vi "lightsource-write.vi"(0 "VISA in":refnum<visa-resource-name>, 2 "set parameters":bool, 3 "NKT Input":T2={"Emission"=FALSE, "Operation Mode"=FALSE, "Power Level"=5.0, "Feedback Level"=0.0, "Short Wavelength (nm)"=560.0, "Long Wavelength (nm)"=580.0, "UV Wavelength (nm)"=400.0} {"UV Wavelength (nm)" min=350.0 max=480.0 step=1.0 format="%.1f"; "Long Wavelength (nm)" min=400.0 max=850.0 step=0.5 format="%.1f"; "Short Wavelength (nm)" min=400.0 max=850.0 step=0.5 format="%.1f"; "Feedback Level" min=0.0 max=90.0 step=0.1 format="%.1f%%"; "Power Level" min=5.0 max=100.0 step=0.1 format="%.1f%%"}) -> (1 "VISA out":refnum<visa-resource-name>, 4 "NKT Output":T1 {"UV Wavelength (nm)" format="%.1f"; "Long Wavelength (nm)" format="%.1f"; "Short Wavelength (nm)" format="%.1f"; "Feedback Level" format="%.1f%%"; "Power Level" format="%.1f%%"; "Temp (°C)" format="%.1f"}, 8 "External Control Cluster":T3)   [LabVIEW 2015]
panel:
  out "Emission on?":bool
  out "Long Wavelength":i32
  out "Short Wavelength":i32
  out "Power Level":i32
  out "Operation Mode":i32
  out "Feedback Level":i32
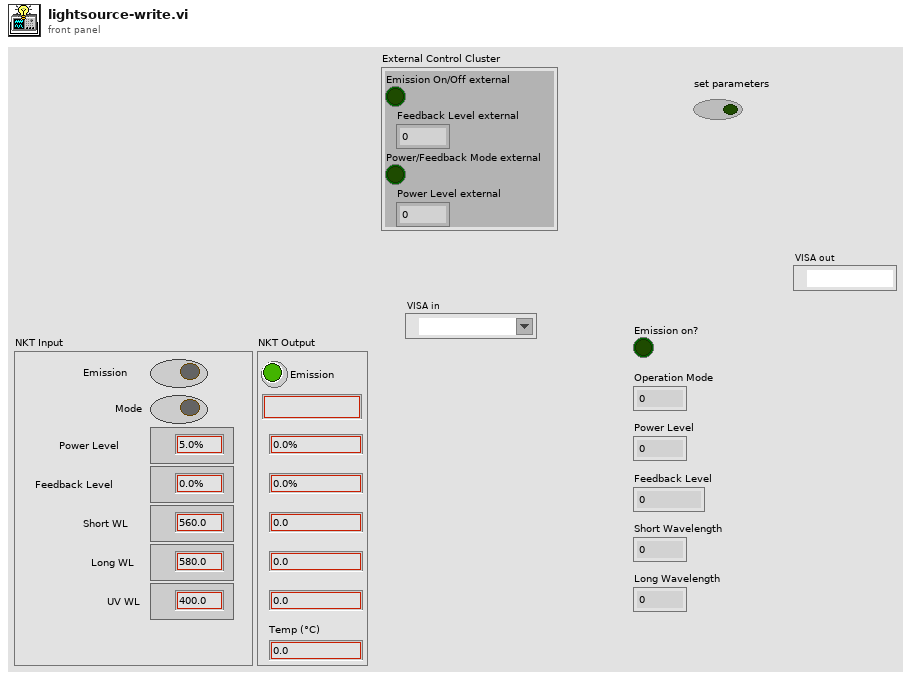
[diagram p1: front panel]
types:
  T1 = cluster{"Emission":bool, "Operation Mode":string, "Power Level":dbl, "Feedback Level":dbl, "Short Wavelength (nm)":dbl, "Long Wavelength (nm)":dbl, "UV Wavelength (nm)":dbl, "Temp (°C)":dbl}
  T2 = cluster{"Emission":bool, "Operation Mode":bool, "Power Level":dbl, "Feedback Level":dbl, "Short Wavelength (nm)":dbl, "Long Wavelength (nm)":dbl, "UV Wavelength (nm)":dbl}
  T3 = cluster{"Emission On/Off external":bool, "Feedback Level external":dbl, "Power/Feedback Mode external":bool, "Power Level external":dbl}
  T4 = cluster{"OpenPort":bool, "ClosePort":bool, "Baudrate":i32, "Wait":u16, "ReadWrite":bool}
  T5 = cluster{"Destination":u8, "Source":u8, "Register":u8, "Array":i16[], "WriteNotRead":bool, "ReadWithPreample":bool, "Ring":u16, "String":string, "Long":i32}
  T6 = cluster{"Source":u8, "TelegramType":u8, "Register":u8, "Destination":u8, "TelegramReceived":bool, "CRC error":bool, "PayloadByteArray":u8[], "(hi.lo)":u16, "Crc16":u16, "Long":i32, "PayloadIntArray":u16[], "String":string}
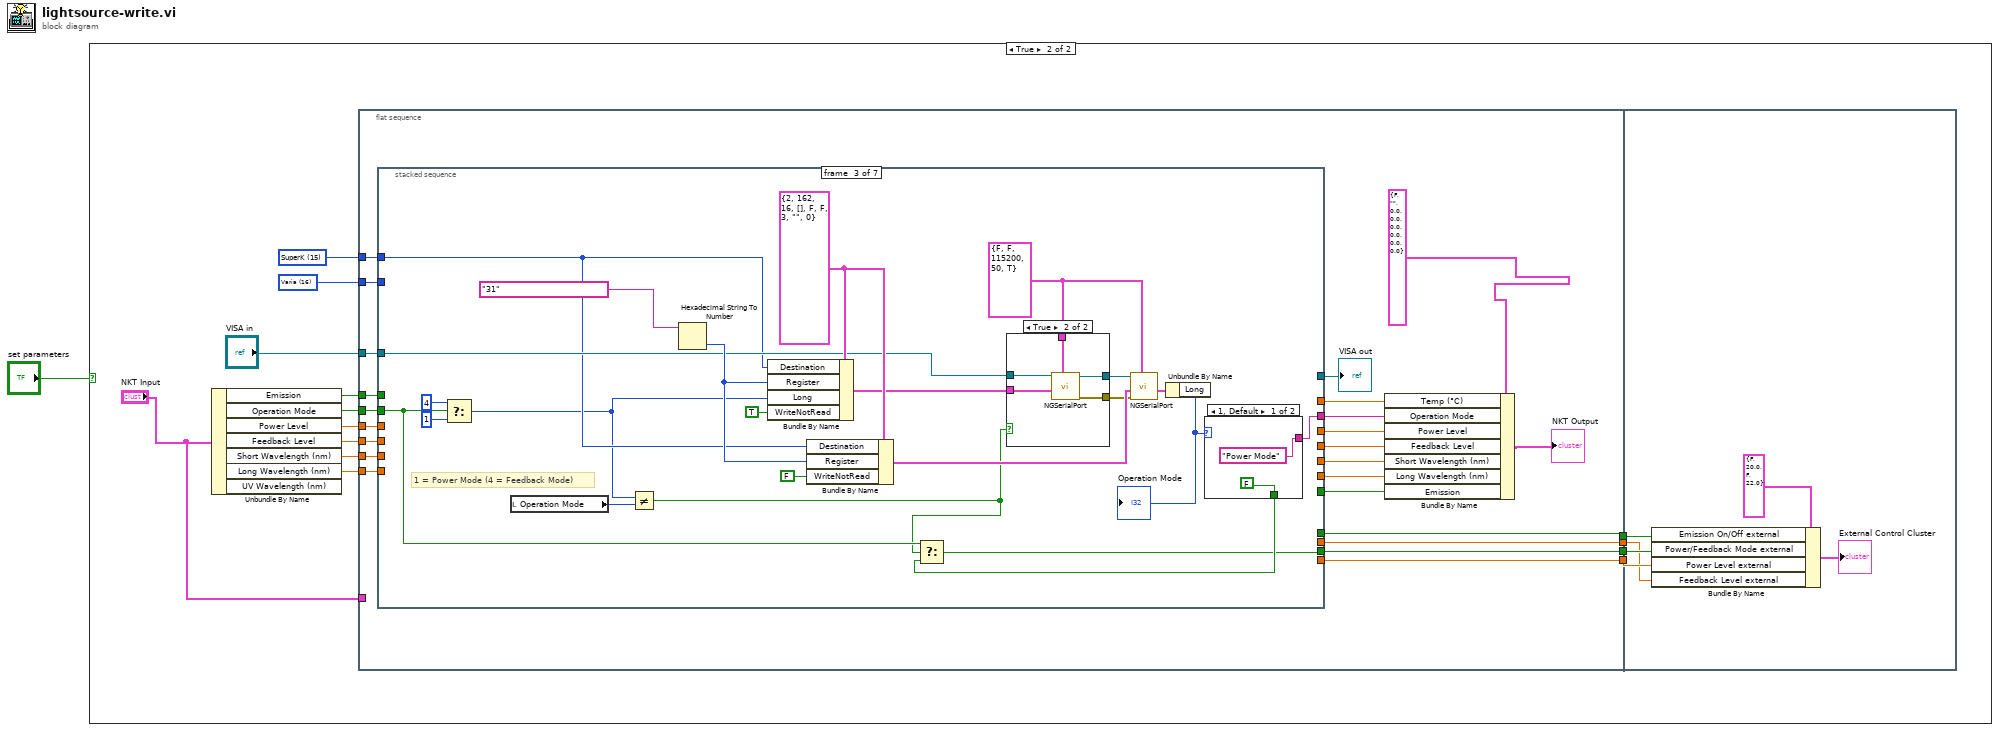
[diagram p0: block diagram]
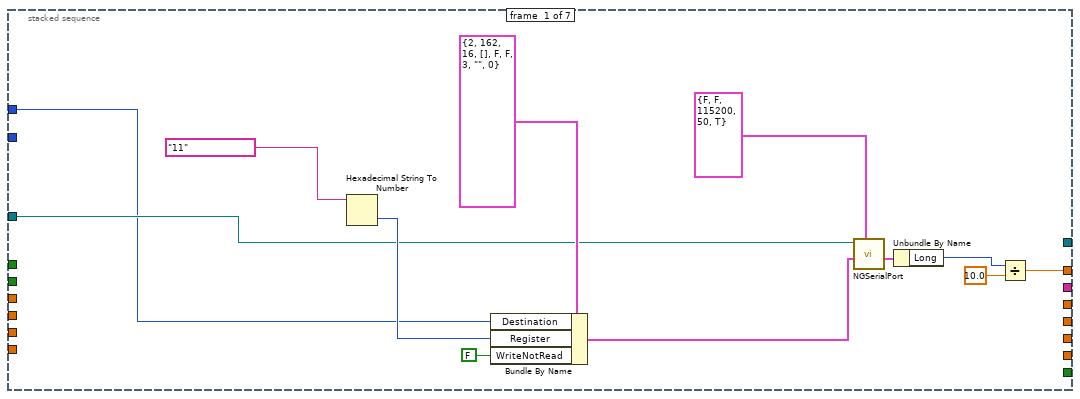
[diagram p3: hidden frame]
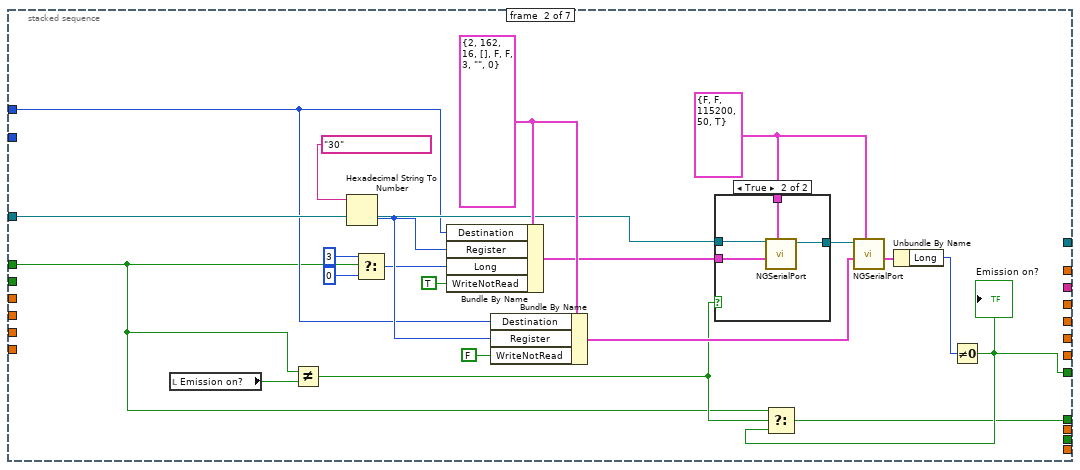
[diagram p4: hidden frame]
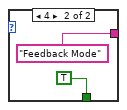
[diagram p6: hidden frame]
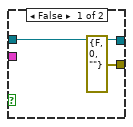
[diagram p7: hidden frame]
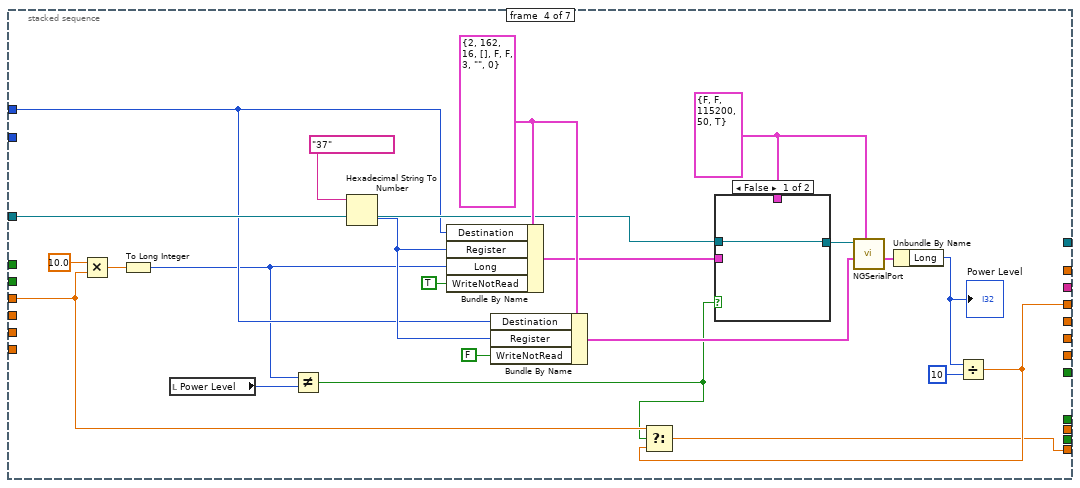
[diagram p8: hidden frame]
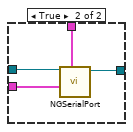
[diagram p9: hidden frame]
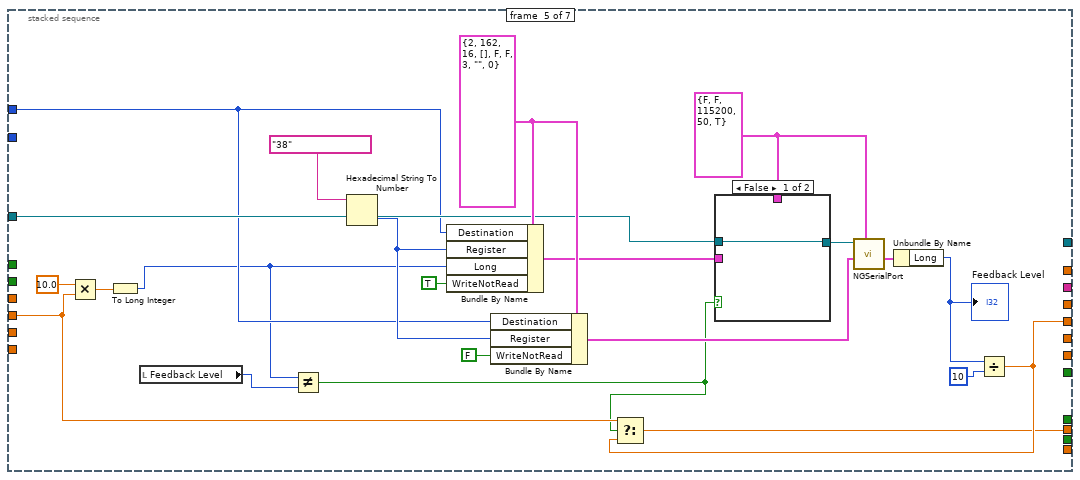
[diagram p10: hidden frame]
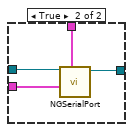
[diagram p11: hidden frame]
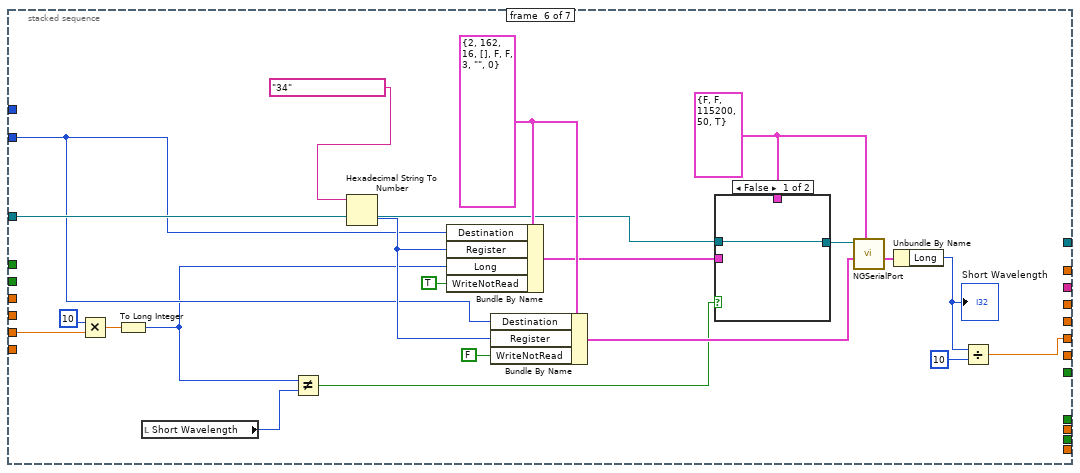
[diagram p12: hidden frame]
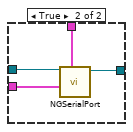
[diagram p13: hidden frame]
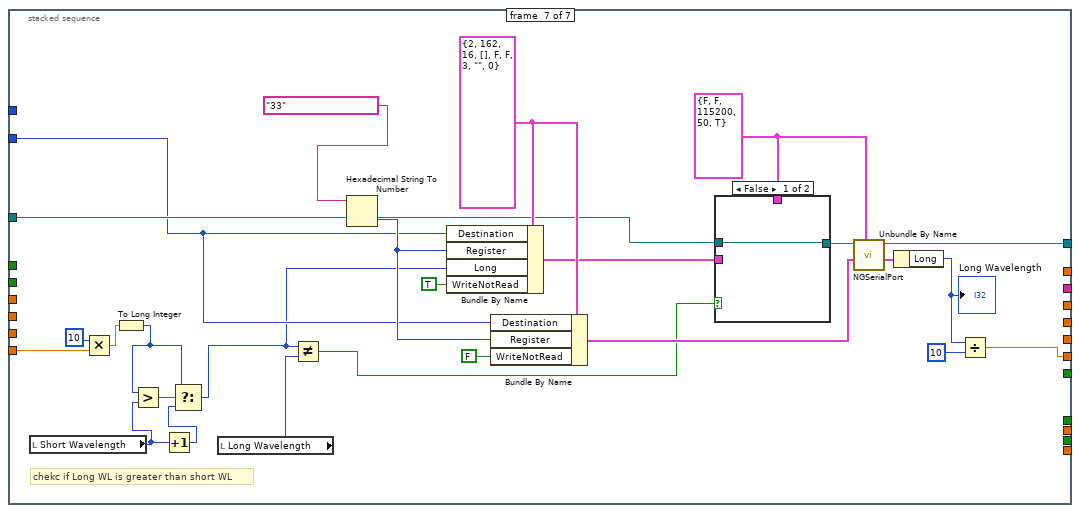
[diagram p14: hidden frame]
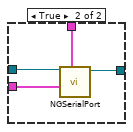
[diagram p15: hidden frame]
diagram:
  n1 = case shown="True" "set parameters" {
    frame False {
    }
    frame True {
      w3 = u16 15 items=["SuperK"=15, "Varia"=16, "UV"=30] ("Module 9")
      w4 = u16 16 items=["SuperK"=15, "Varia"=16, "UV"=30] ("Module 9")
      n2 = Unbundle By Name("NKT Input") -> ("Emission"=w10:bool, "Operation Mode"=w9:bool, "Power Level"=w8:dbl, "Feedback Level"=w7:dbl, "Short Wavelength (nm)"=w6:dbl, "Long Wavelength (nm)"=w5:dbl)  [unwired: 1 out]
      n3 = flat-sequence {
        tunnel: "VISA in" -> [w38]
        tunnel: w3 -> [w36]
        tunnel: w4 -> [w35]
        tunnel: w10 -> [w34]
        tunnel: w9 -> [w33]
        tunnel: w8 -> [w32]
        tunnel: w7 -> [w31]
        tunnel: w6 -> [w30]
        tunnel: w5 -> [w29]
        tunnel: "NKT Input" -> [_]
        tunnel: [w22] -> w15
        tunnel: [w21] -> w14
        tunnel: [w20] -> w13
        tunnel: [w19] -> w12
        tunnel: w15 -> [w226]
        tunnel: w14 -> [w225]
        tunnel: w13 -> [w224]
        tunnel: w12 -> [w227]
        frame #0 {
          n4 = stacked-sequence {
            tunnel: w38 -> [w43 w61 w89 w122 w148 w176 w207]
            tunnel: [_ _ _ _ _ _ w198] -> w37
            tunnel: w36 -> [w42 w60 w88 w121 w147 _ _]
            tunnel: w35 -> [_ _ _ _ _ w175 w206]
            tunnel: [w39 _ _ _ _ _ _] -> w28
            tunnel: w34 -> [_ w54 _ _ _ _ _]
            tunnel: [_ w57 _ _ _ _ _] -> w18
            tunnel: w33 -> [_ _ w81 _ _ _ _]
            tunnel: [_ _ w83 _ _ _ _] -> w27
            tunnel: w32 -> [_ _ _ w114 _ _ _]
            tunnel: [_ _ _ w113 _ _ _] -> w26
            tunnel: w31 -> [_ _ _ _ w141 _ _]
            tunnel: w30 -> [_ _ _ _ _ w169 _]
            tunnel: w29 -> [_ _ _ _ _ _ w200]
            tunnel: [_ _ _ _ w140 _ _] -> w25
            tunnel: [_ _ _ _ _ w165 _] -> w24
            tunnel: [_ _ _ _ _ _ w191] -> w23
            tunnel: [_ _ w79 _ _ _ _] -> w22
            tunnel: [_ _ _ w112 _ _ _] -> w21
            tunnel: [_ _ _ _ w139 _ _] -> w20
            tunnel: [_ w56 _ _ _ _ _] -> w19
            frame #0 {
              n5 = Hexadecimal String To Number(string="11" ("Super K Register 4")) -> (number=w48:u32)  [unwired: 2 in, 1 out]
              n6 = Bundle By Name(cluster=T5 {"Destination"=2, "Source"=162, "Register"=16, "Array"=[], "WriteNotRead"=FALSE, "ReadWithPreample"=FALSE, "Ring"=3, "String"="", "Long"=0} ("InParameters"), "Destination"=w42, "Register"=w48, "WriteNotRead"=FALSE) -> (w47:T5)
              n7 = call "NGSerialPort.vi"("PortParameters"=T4 {"OpenPort"=FALSE, "ClosePort"=FALSE, "Baudrate"=115200, "Wait"=50, "ReadWrite"=TRUE}, "InParameters"=w47, "VISA in"=w43) -> ("OutParameters"=w49:T6)  [unwired: 6 in, 2 out]
              n8 = Unbundle By Name(w49) -> ("Long"=w40:i32)
              n9 = Divide(x=w40, y=10.0) -> (x/y=w39:dbl)
            }
            frame #1 {
              w65 = T4 {"OpenPort"=FALSE, "ClosePort"=FALSE, "Baudrate"=115200, "Wait"=50, "ReadWrite"=TRUE} ("PortParameters")
              w66 = T5 {"Destination"=2, "Source"=162, "Register"=16, "Array"=[], "WriteNotRead"=FALSE, "ReadWithPreample"=FALSE, "Ring"=3, "String"="", "Long"=0} ("InParameters")
              n10 = local read "Emission on?"() -> (w58:bool)
              n11 = Not Equal?(x=w54, y=w58) -> (x != y?=w55:bool)
              n12 = Hexadecimal String To Number(string="30" ("Super K Register 5")) -> (number=w69:u32)  [unwired: 2 in, 1 out]
              n13 = Select(t=3, s=w54, f=0) -> (s? t:f=w52:i32)
              n14 = Bundle By Name(cluster=w66, "Destination"=w60, "Register"=w69, "Long"=w52, "WriteNotRead"=TRUE) -> (w62:T5)
              n15 = Bundle By Name(cluster=w66, "Destination"=w60, "Register"=w69, "WriteNotRead"=FALSE) -> (w68:T5)
              n16 = case shown="True" w55 {
                tunnel: w62 -> [_ w76]
                tunnel: w61 -> [w72 w75]
                tunnel: [w72 w74] -> w64
                tunnel: w65 -> [_ w73]
                frame False {
                }
                frame True {
                  n17 = call "NGSerialPort.vi"("PortParameters"=w73, "InParameters"=w76, "VISA in"=w75) -> ("VISA out"=w74:refnum<visa-resource-name>)  [unwired: 6 in, 2 out]
                }
              }
              n18 = call "NGSerialPort.vi"("PortParameters"=w65, "InParameters"=w68, "VISA in"=w64) -> ("OutParameters"=w70:T6)  [unwired: 6 in, 2 out]
              n19 = Unbundle By Name(w70) -> ("Long"=w59:i32)
              n20 = Not Equal To 0?(x=w59) -> (x != 0?=w57:bool)
              "Emission on?" <- w57
              n21 = Select(t=w54, s=w55, f=w57) -> (s? t:f=w56:bool)
            }
            frame #2 {
              w93 = T4 {"OpenPort"=FALSE, "ClosePort"=FALSE, "Baudrate"=115200, "Wait"=50, "ReadWrite"=TRUE} ("PortParameters")
              w94 = T5 {"Destination"=2, "Source"=162, "Register"=16, "Array"=[], "WriteNotRead"=FALSE, "ReadWithPreample"=FALSE, "Ring"=3, "String"="", "Long"=0} ("InParameters")
              # "1 = Power Mode (4 = Feedback Mode)"
              n22 = Select(t=4, s=w81, f=1) -> (s? t:f=w85:i32)
              n23 = local read "Operation Mode"() -> (w82:i32)
              n24 = Not Equal?(x=w85, y=w82) -> (x != y?=w78:bool)
              n25 = Hexadecimal String To Number(string="31" ("Super K Register 6")) -> (number=w97:u32)  [unwired: 2 in, 1 out]
              n26 = Bundle By Name(cluster=w94, "Destination"=w88, "Register"=w97, "Long"=w85, "WriteNotRead"=TRUE) -> (w90:T5)
              n27 = Bundle By Name(cluster=w94, "Destination"=w88, "Register"=w97, "WriteNotRead"=FALSE) -> (w96:T5)
              n28 = case shown="True" w78 {
                tunnel: w90 -> [_ w110]
                tunnel: w89 -> [w105 w109]
                tunnel: [w105 w108] -> w92
                tunnel: w93 -> [_ w107]
                tunnel: [errorcluster {"status"=FALSE, "code"=0, "source"=""} ("error out") w106] -> w77
                frame False {
                }
                frame True {
                  n29 = call "NGSerialPort.vi"("PortParameters"=w107, "InParameters"=w110, "VISA in"=w109) -> ("error out"=w106:errorcluster, "VISA out"=w108:refnum<visa-resource-name>)  [unwired: 6 in, 1 out]
                }
              }
              n30 = call "NGSerialPort.vi"("PortParameters"=w93, "error in"=w77, "InParameters"=w96, "VISA in"=w92) -> ("OutParameters"=w98:T6)  [unwired: 5 in, 2 out]
              n31 = Unbundle By Name(w98) -> ("Long"=w84:i32)
              "Operation Mode" <- w84
              n32 = case shown="1, Default" w84 {
                tunnel: ["Power Mode" ("Operation Mode 2") "Feedback Mode" ("Operation Mode 2")] -> w83
                tunnel: [FALSE TRUE] -> w80
                frame 1, Default {
                }
                frame 4 {
                }
              }
              n33 = Select(t=w81, s=w78, f=w80) -> (s? t:f=w79:bool)
            }
            frame #3 {
              w126 = T4 {"OpenPort"=FALSE, "ClosePort"=FALSE, "Baudrate"=115200, "Wait"=50, "ReadWrite"=TRUE} ("PortParameters")
              w127 = T5 {"Destination"=2, "Source"=162, "Register"=16, "Array"=[], "WriteNotRead"=FALSE, "ReadWithPreample"=FALSE, "Ring"=3, "String"="", "Long"=0} ("InParameters")
              n34 = Multiply(x=10.0, y=w114) -> (x*y=w119:dbl)
              n35 = To Long Integer(number=w119) -> (32bit integer=w118:i32)
              n36 = local read "Power Level"() -> (w116:i32)
              n37 = Not Equal?(x=w118, y=w116) -> (x != y?=w111:bool)
              n38 = Hexadecimal String To Number(string="37" ("Super K Register 7")) -> (number=w130:u32)  [unwired: 2 in, 1 out]
              n39 = Bundle By Name(cluster=w127, "Destination"=w121, "Register"=w130, "Long"=w118, "WriteNotRead"=TRUE) -> (w123:T5)
              n40 = Bundle By Name(cluster=w127, "Destination"=w121, "Register"=w130, "WriteNotRead"=FALSE) -> (w129:T5)
              n41 = case shown="False" w111 {
                tunnel: w123 -> [_ w137]
                tunnel: w122 -> [w133 w136]
                tunnel: [w133 w135] -> w125
                tunnel: w126 -> [_ w134]
                frame False {
                }
                frame True {
                  n42 = call "NGSerialPort.vi"("PortParameters"=w134, "InParameters"=w137, "VISA in"=w136) -> ("VISA out"=w135:refnum<visa-resource-name>)  [unwired: 6 in, 2 out]
                }
              }
              n43 = call "NGSerialPort.vi"("PortParameters"=w126, "InParameters"=w129, "VISA in"=w125) -> ("OutParameters"=w131:T6)  [unwired: 6 in, 2 out]
              n44 = Unbundle By Name(w131) -> ("Long"=w117:i32)
              "Power Level" <- w117
              n45 = Divide(x=w117, y=10) -> (x/y=w113:dbl)
              n46 = Select(t=w114, s=w111, f=w113) -> (s? t:f=w112:dbl)
            }
            frame #4 {
              w153 = T4 {"OpenPort"=FALSE, "ClosePort"=FALSE, "Baudrate"=115200, "Wait"=50, "ReadWrite"=TRUE} ("PortParameters")
              w154 = T5 {"Destination"=2, "Source"=162, "Register"=16, "Array"=[], "WriteNotRead"=FALSE, "ReadWithPreample"=FALSE, "Ring"=3, "String"="", "Long"=0} ("InParameters")
              n47 = Multiply(x=10.0, y=w141) -> (x*y=w145:dbl)
              n48 = To Long Integer(number=w145) -> (32bit integer=w144:i32)
              n49 = local read "Feedback Level"() -> (w149:i32)
              n50 = Not Equal?(x=w144, y=w149) -> (x != y?=w138:bool)
              n51 = Hexadecimal String To Number(string="38" ("Super K Register 8")) -> (number=w157:u32)  [unwired: 2 in, 1 out]
              n52 = Bundle By Name(cluster=w154, "Destination"=w147, "Register"=w157, "Long"=w144, "WriteNotRead"=TRUE) -> (w150:T5)
              n53 = Bundle By Name(cluster=w154, "Destination"=w147, "Register"=w157, "WriteNotRead"=FALSE) -> (w156:T5)
              n54 = case shown="False" w138 {
                tunnel: w150 -> [_ w164]
                tunnel: w148 -> [w160 w163]
                tunnel: [w160 w162] -> w152
                tunnel: w153 -> [_ w161]
                frame False {
                }
                frame True {
                  n55 = call "NGSerialPort.vi"("PortParameters"=w161, "InParameters"=w164, "VISA in"=w163) -> ("VISA out"=w162:refnum<visa-resource-name>)  [unwired: 6 in, 2 out]
                }
              }
              n56 = call "NGSerialPort.vi"("PortParameters"=w153, "InParameters"=w156, "VISA in"=w152) -> ("OutParameters"=w158:T6)  [unwired: 6 in, 2 out]
              n57 = Unbundle By Name(w158) -> ("Long"=w143:i32)
              "Feedback Level" <- w143
              n58 = Divide(x=w143, y=10) -> (x/y=w140:dbl)
              n59 = Select(t=w141, s=w138, f=w140) -> (s? t:f=w139:dbl)
            }
            frame #5 {
              w180 = T4 {"OpenPort"=FALSE, "ClosePort"=FALSE, "Baudrate"=115200, "Wait"=50, "ReadWrite"=TRUE} ("PortParameters")
              w181 = T5 {"Destination"=2, "Source"=162, "Register"=16, "Array"=[], "WriteNotRead"=FALSE, "ReadWithPreample"=FALSE, "Ring"=3, "String"="", "Long"=0} ("InParameters")
              n60 = Multiply(x=10, y=w169) -> (x*y=w167:dbl)
              n61 = To Long Integer(number=w167) -> (32bit integer=w166:i32)
              n62 = local read "Short Wavelength"() -> (w170:i32)
              n63 = Not Equal?(x=w166, y=w170) -> (x != y?=w168:bool)
              n64 = Hexadecimal String To Number(string="34" ("Varia Register 13")) -> (number=w184:u32)  [unwired: 2 in, 1 out]
              n65 = Bundle By Name(cluster=w181, "Destination"=w175, "Register"=w184, "Long"=w166, "WriteNotRead"=TRUE) -> (w177:T5)
              n66 = Bundle By Name(cluster=w181, "Destination"=w175, "Register"=w184, "WriteNotRead"=FALSE) -> (w183:T5)
              n67 = case shown="False" w168 {
                tunnel: w177 -> [_ w190]
                tunnel: w176 -> [w186 w189]
                tunnel: [w186 w188] -> w179
                tunnel: w180 -> [_ w187]
                frame False {
                }
                frame True {
                  n68 = call "NGSerialPort.vi"("PortParameters"=w187, "InParameters"=w190, "VISA in"=w189) -> ("VISA out"=w188:refnum<visa-resource-name>)  [unwired: 6 in, 2 out]
                }
              }
              n69 = call "NGSerialPort.vi"("PortParameters"=w180, "InParameters"=w183, "VISA in"=w179) -> ("OutParameters"=w185:T6)  [unwired: 6 in, 2 out]
              n70 = Unbundle By Name(w185) -> ("Long"=w171:i32)
              "Short Wavelength" <- w171
              n71 = Divide(x=w171, y=10 ("x")) -> (x/y=w165:dbl)
            }
            frame #6 {
              w211 = T4 {"OpenPort"=FALSE, "ClosePort"=FALSE, "Baudrate"=115200, "Wait"=50, "ReadWrite"=TRUE} ("PortParameters")
              w212 = T5 {"Destination"=2, "Source"=162, "Register"=16, "Array"=[], "WriteNotRead"=FALSE, "ReadWithPreample"=FALSE, "Ring"=3, "String"="", "Long"=0} ("InParameters")
              # "chekc if Long WL is greater than short WL"
              n72 = local read "Short Wavelength"() -> (w196:i32)
              n73 = Multiply(x=10, y=w200) -> (x*y=w193:dbl)
              n74 = To Long Integer(number=w193) -> (32bit integer=w192:i32)
              n75 = Greater?(x=w192, y=w196) -> (0:w197:bool)
              n76 = Increment(x=w196) -> (x+1=w195:i32)
              n77 = Select(t=w192, s=w197, f=w195) -> (s? t:f=w194:i32)
              n78 = local read "Long Wavelength"() -> (w201:i32)
              n79 = Not Equal?(x=w194, y=w201) -> (x != y?=w199:bool)
              n80 = Hexadecimal String To Number(string="33" ("Varia Register 12")) -> (number=w215:u32)  [unwired: 2 in, 1 out]
              n81 = Bundle By Name(cluster=w212, "Destination"=w206, "Register"=w215, "Long"=w194, "WriteNotRead"=TRUE) -> (w208:T5)
              n82 = Bundle By Name(cluster=w212, "Destination"=w206, "Register"=w215, "WriteNotRead"=FALSE) -> (w214:T5)
              n83 = case shown="False" w199 {
                tunnel: w208 -> [_ w221]
                tunnel: w207 -> [w217 w220]
                tunnel: [w217 w219] -> w210
                tunnel: w211 -> [_ w218]
                frame False {
                }
                frame True {
                  n84 = call "NGSerialPort.vi"("PortParameters"=w218, "InParameters"=w221, "VISA in"=w220) -> ("VISA out"=w219:refnum<visa-resource-name>)  [unwired: 6 in, 2 out]
                }
              }
              n85 = call "NGSerialPort.vi"("PortParameters"=w211, "InParameters"=w214, "VISA in"=w210) -> ("OutParameters"=w216:T6, "VISA out"=w198:refnum<visa-resource-name>)  [unwired: 6 in, 1 out]
              n86 = Unbundle By Name(w216) -> ("Long"=w202:i32)
              "Long Wavelength" <- w202
              n87 = Divide(x=w202, y=10 ("x")) -> (x/y=w191:dbl)
            }
          }
          "VISA out" <- w37
          n88 = Bundle By Name(cluster=T1 {"Emission"=FALSE, "Operation Mode"="", "Power Level"=0.0, "Feedback Level"=0.0, "Short Wavelength (nm)"=0.0, "Long Wavelength (nm)"=0.0, "UV Wavelength (nm)"=0.0, "Temp (°C)"=0.0} ("NKT Output"), "Temp (°C)"=w28, "Operation Mode"=w27, "Power Level"=w26, "Feedback Level"=w25, "Short Wavelength (nm)"=w24, "Long Wavelength (nm)"=w23, "Emission"=w18) -> (→"NKT Output":T1)
        }
        frame #1 {
          n89 = Bundle By Name(cluster=T3 {"Emission On/Off external"=FALSE, "Feedback Level external"=20.0, "Power/Feedback Mode external"=FALSE, "Power Level external"=22.0} ("External Control Cluster 2"), "Emission On/Off external"=w227, "Power/Feedback Mode external"=w226, "Power Level external"=w225, "Feedback Level external"=w224) -> (→"External Control Cluster":T3)
        }
      }
    }
  }
